vi "ThrowTile.vi"(1 "HandSize":u16, 2 "Hand":u16[](array[ring])) -> (0 "Which":u16)   [LabVIEW 2025]
panel:
  out "Min":i16
  out "Temp":u16[](array[numeric])
  out "HandCount":u16[](array[numeric])
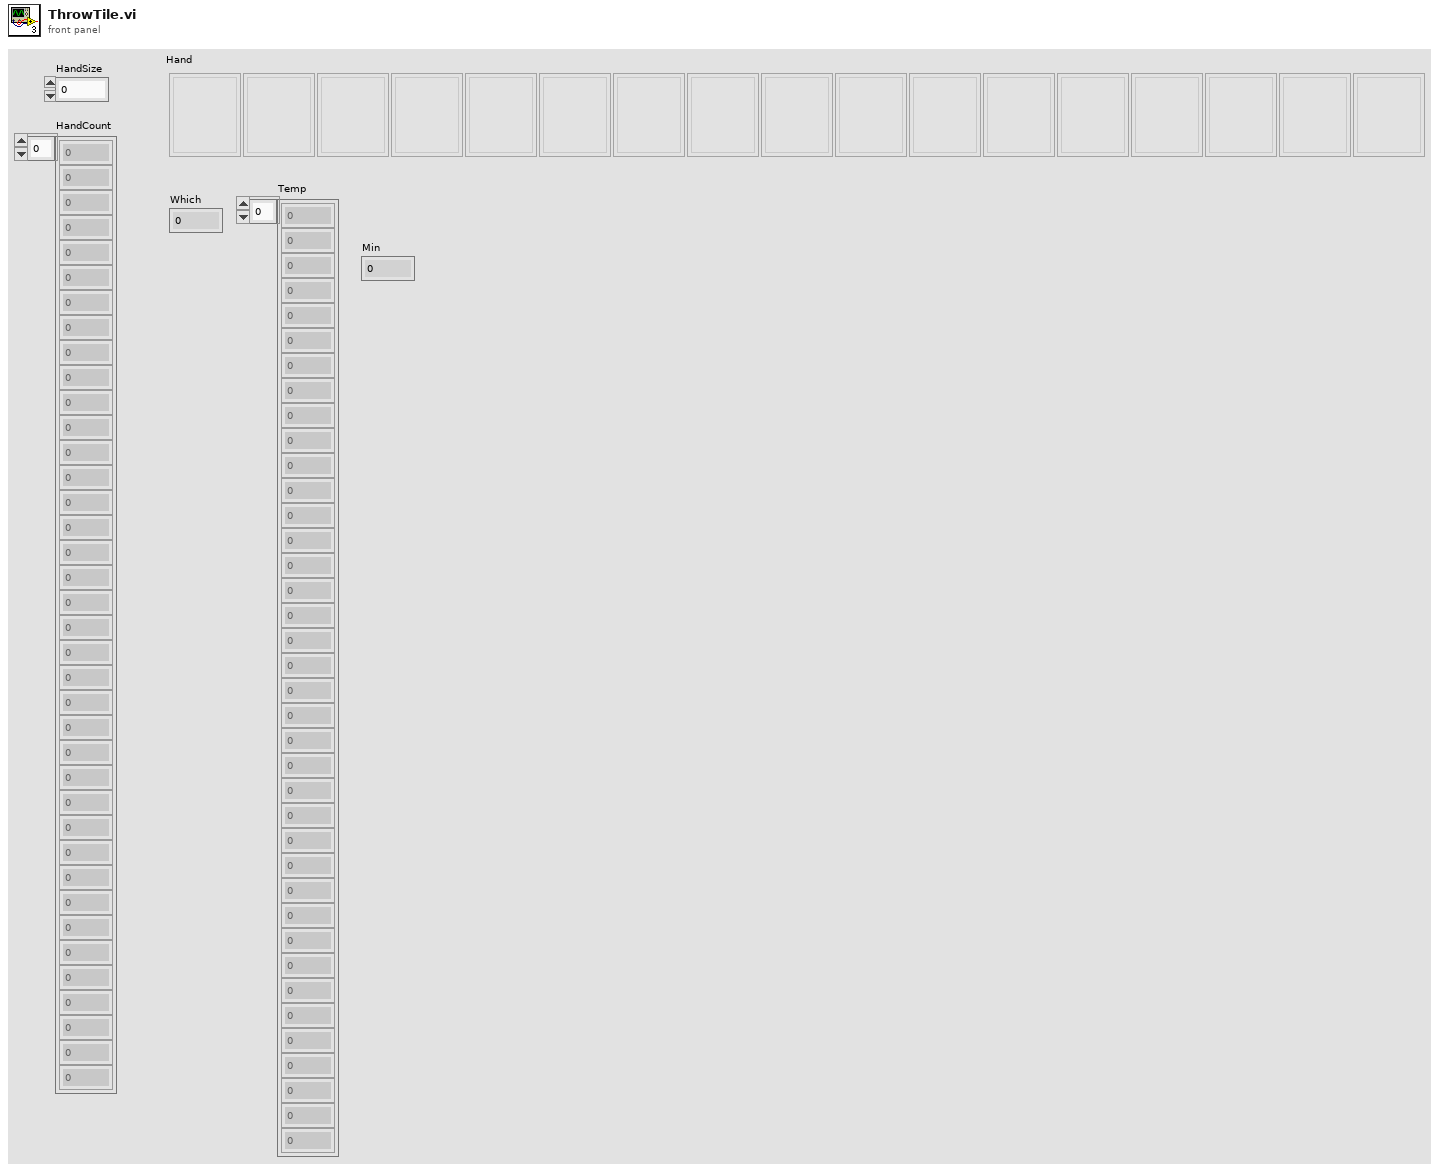
[diagram p1: front panel]
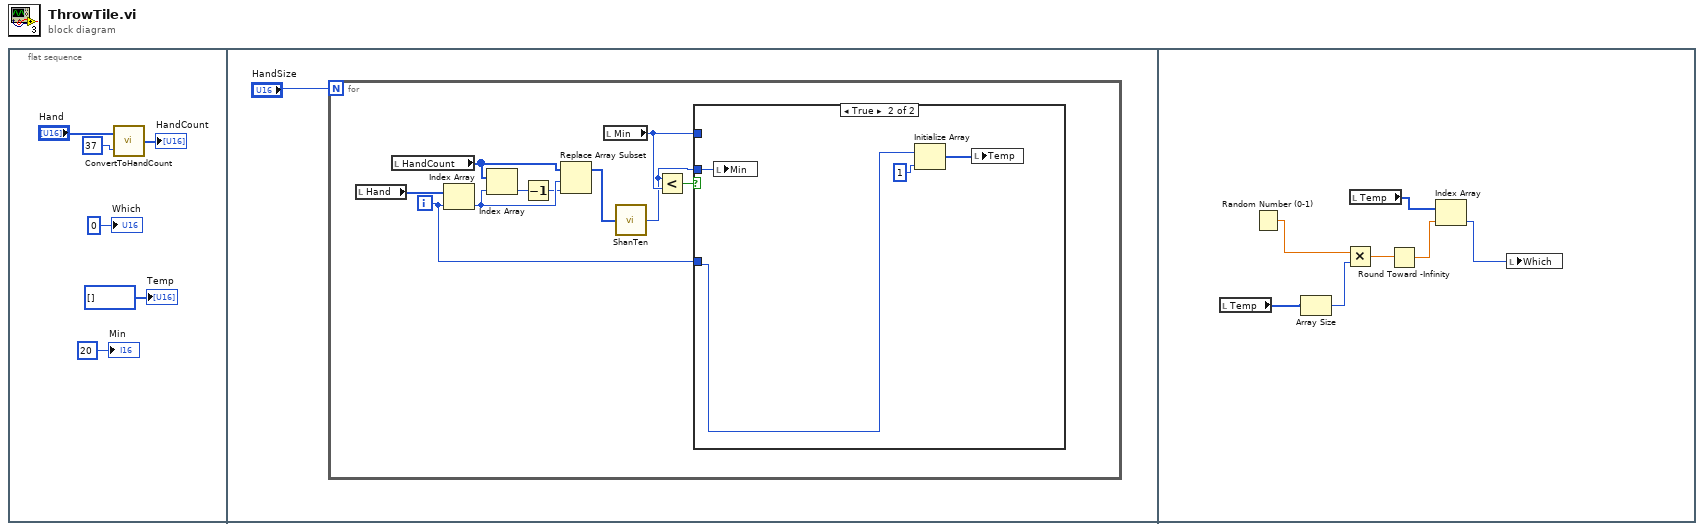
[diagram p0: block diagram]
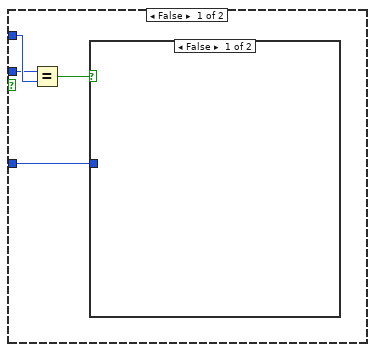
[diagram p2: hidden frame]
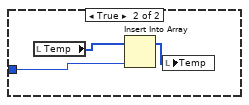
[diagram p3: hidden frame]
diagram:
  n1 = flat-sequence {
    frame #0 {
      n2 = call "ConvertToHandCount.vi"("AddtionalTile"=u16 37, "Hand"="Hand") -> ("HandCount"=→"HandCount":u16[])
      "Which" <- u16 0 ("Which")
      "Temp" <- u16[] [] ("Temp")
      "Min" <- u16 20 ("Max")
    }
    frame #1 {
      n3 = for {
        N: "HandSize" -> [_]
        i -> [w10]
        n4 = local read "Hand"() -> (w17:u16[])
        n5 = local read "HandCount"() -> (w15:u16[])
        n6 = Index Array(array=w17, index=w10) -> (element=w14:u16)
        n7 = Index Array(array=w15, index=w14) -> (element=w16:u16)
        n8 = Decrement(x=w16) -> (x-1=w13:u16)
        n9 = Replace Array Subset(array=w15, new element=w13, index=w14) -> (w9:u16[])
        n10 = local read "Min"() -> (w11:i16)
        n11 = call "ShanTen.vi"("Count"=w9) -> ("ShanTen"=w8:i16)
        n12 = Less?(x=w8, y=w11) -> (x < y?=w12:bool)
        n13 = case shown="True" w12 {
          tunnel: w8 -> [w19 w28]
          tunnel: w11 -> [w21 _]
          tunnel: w10 -> [w18 w25]
          frame False {
            n14 = Equal?(x=w19, y=w21) -> (x = y?=w20:bool)
            n15 = case shown="False" w20 {
              tunnel: w18 -> [_ w22]
              frame False {
              }
              frame True {
                n16 = local read "Temp"() -> (w23:u16[])
                n17 = Insert Into Array(array=w23, new element=w22) -> (w24:u16[])  [unwired: 1 in]
                n18 = local write "Temp"(w24) -> ()
              }
            }
          }
          frame True {
            n19 = local write "Min"(w28) -> ()
            n20 = Initialize Array(w25, 1) -> (w27:i32[])
            n21 = local write "Temp"(w27) -> ()
          }
        }
      }
    }
    frame #2 {
      n22 = local read "Temp"() -> (w29:u16[])
      n23 = Random Number (0-1)() -> (number: 0 to 1=w35:dbl)
      n24 = Array Size(array=w29) -> (size(s)=w30:i32)
      n25 = Multiply(x=w35, y=w30) -> (x*y=w34:dbl)
      n26 = local read "Temp"() -> (w33:u16[])
      n27 = Round Toward -Infinity(1:w34) -> (0:w32:dbl)
      n28 = Index Array(array=w33, index=w32) -> (element=w31:u16)
      n29 = local write "Which"(w31) -> ()
    }
  }
